vi "Check for Buffer Request.vi"(8 "error in (no error)":errorcluster, 9 "timeout ms (25000)":i32, 11 "connection ID in":refnum<k5>) -> (0 "error out":errorcluster, 1 "timed out?":bool, 2 "buffer descriptor":T1, 3 "connection ID out":refnum<k5>)   [LabVIEW 2021, in "DSF Core.lvlib" / "Data Server Thread.lvclass"]
uses:
  Data Server Thread.lvclass
  DSF Buffer Subset Descriptor.ctl
  Typedefs/DSF Buffer Type.ctl
  DSF Core.lvlib
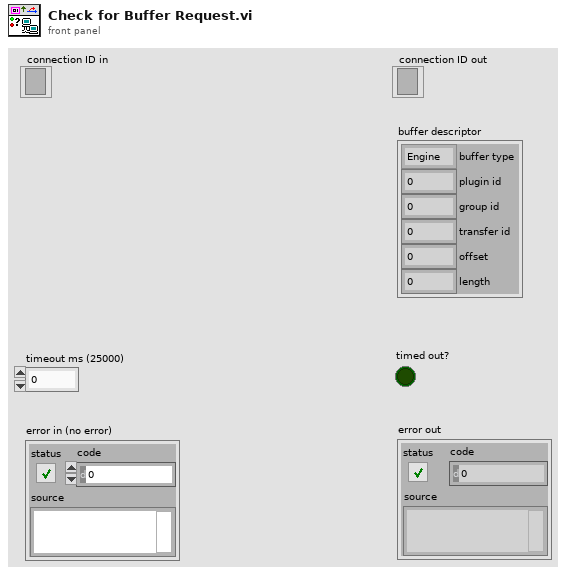
[diagram p1: front panel]
types:
  T1 = typedef "DSF Core.lvlib/DSF Buffer Subset Descriptor.ctl" = cluster{"buffer type":T2, "plugin id":i32, "group id":i32, "transfer id":i32, "offset":u64, "length":i64}
  T2 = typedef "DSF Core.lvlib/DSF Buffer Type.ctl" = enum16{"Engine", "String"}
  T3 = enum16{"big-endian, network order", "native, host order", "little-endian"}
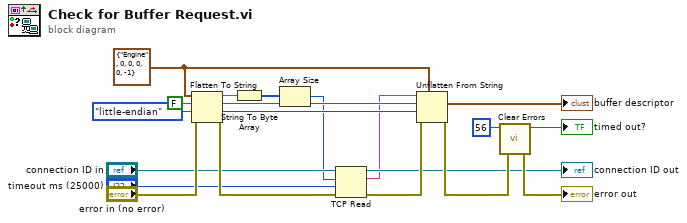
[diagram p0: block diagram]
diagram:
  w4 = T3."little-endian" ("byte order (0:big-endian, network order)")
  w3 = FALSE ("prepend array or string size? (T)")
  w12 = T1 {"buffer type"=enum."Engine", "plugin id"=0, "group id"=0, "transfer id"=0, "offset"=0, "length"=-1} ("Cluster")
  n1 = Flatten To String(anything=w12, prepend array or string size? (T)=w3, byte order (0:big-endian, network order)=w4, error in (no error)="error in (no error)") -> (data string=w16:string, error out=w17:errorcluster)  [unwired: 1 out]
  n2 = String To Byte Array(string=w16) -> (unsigned byte array=w15:u8[])
  n3 = Array Size(array=w15) -> (size(s)=w2:i32)
  n4 = TCP Read(connection ID="connection ID in", bytes to read=w2, error in (no error)=w17, 9:"timeout ms (25000)") -> (connection ID out=→"connection ID out":refnum<k5>, data out=w1:string, error out=w13:errorcluster)  [unwired: 1 in]
  n5 = Unflatten From String(type=w12, binary string=w1, data includes array or string size? (T)=w3, byte order (0:big-endian, network order)=w4, error in (no error)=w13) -> (value=→"buffer descriptor":T1, error out=w9:errorcluster)  [unwired: 1 out]
  n6 = call <vilib>:"Clear Errors.vi"("error in (no error)"=w9, "specific error code to clear (0: all)"=56) -> ("error out"=→"error out":errorcluster, "specific error cleared?"=→"timed out?":bool)  [unwired: 4 in]
